vi "CD Init_Prepare Inline Data_Fill In RT part of Frame Descriptor -Broadcast.vi"(8 "RTs In":T1[](array[typedef]) {"Mode Codes"."Words Item Refs" format="%.0x"; "Mode Codes"."Words Block Data Refs"."Data Reference" format="%.0x"; "Mode Codes"."Timestamp Channel Data Reference" format="%.0x"; "subAddresses"."Words Item Refs" format="%.0x"; "subAddresses"."Words Block Data Refs"."Data Reference" format="%.0x"; "subAddresses"."Timestamp Channel Data Reference" format="%.0x"; "Status Channel Data Reference" format="%.0x"; "Command Channels Refs" format="%.0x"}, 11 "message":T10 {"Timestamp Channel Data Reference" format="%.0x"; "Status Channel Data Refs" format="%.0x"; "Words Item Refs" format="%.0x"; "Words Block Data Refs"."Data Reference" format="%.0x"}) -> (0 "RTs Out":T1[](array[typedef]) {"Mode Codes"."Words Item Refs" format="%.0x"; "Mode Codes"."Words Block Data Refs"."Data Reference" format="%.0x"; "Mode Codes"."Timestamp Channel Data Reference" format="%.0x"; "subAddresses"."Words Item Refs" format="%.0x"; "subAddresses"."Words Block Data Refs"."Data Reference" format="%.0x"; "subAddresses"."Timestamp Channel Data Reference" format="%.0x"; "Status Channel Data Reference" format="%.0x"; "Command Channels Refs" format="%.0x"}, 3 "RTs Frame Descriptors":T9[](array[typedef]) {"Status Channel Ref" format="%.0x"; "Words Block Data Refs"."Data Reference" format="%.0x"; "Timestamp Channel Data Reference" format="%.0x"})   [LabVIEW 2017, in "Ballard MIL-1553 Engine.lvlib"]
uses:
  Ballard MIL-1553 Engine.lvlib
  Shared/Controls and Global/RT Message.ctl
  Shared/Controls and Global/RT messageType.ctl
  Shared/Controls and Global/RT CWD1.ctl
  Shared/Controls and Global/RT CWD2.ctl
  <vilib>/NI Veristand/Custom Device API/Data Reference.ctl
  <vilib>/NI Veristand/Custom Device API/Custom Device Item Ref.ctl
  <vilib>/NI Veristand/Custom Device API/Block Data Reference.ctl
  Controls/RT Inline Frame Descriptor_RT.ctl
  Shared/Controls and Global/RT Remote Terminal.ctl
  Shared/Controls and Global/RT Remote Terminal_rtMode.ctl
  Shared/Controls and Global/RT Remote Terminal_RT subAddress.ctl
  Shared/Controls and Global/RT Remote Terminal_RT direction.ctl
  Shared/Controls and Global/RT Remote Terminal_RT Mode Code.ctl
  <vilib>/NI VeriStand/Custom Device API/Custom Device API.lvlib
  Shared/Ballard 1553 Shared.lvlib
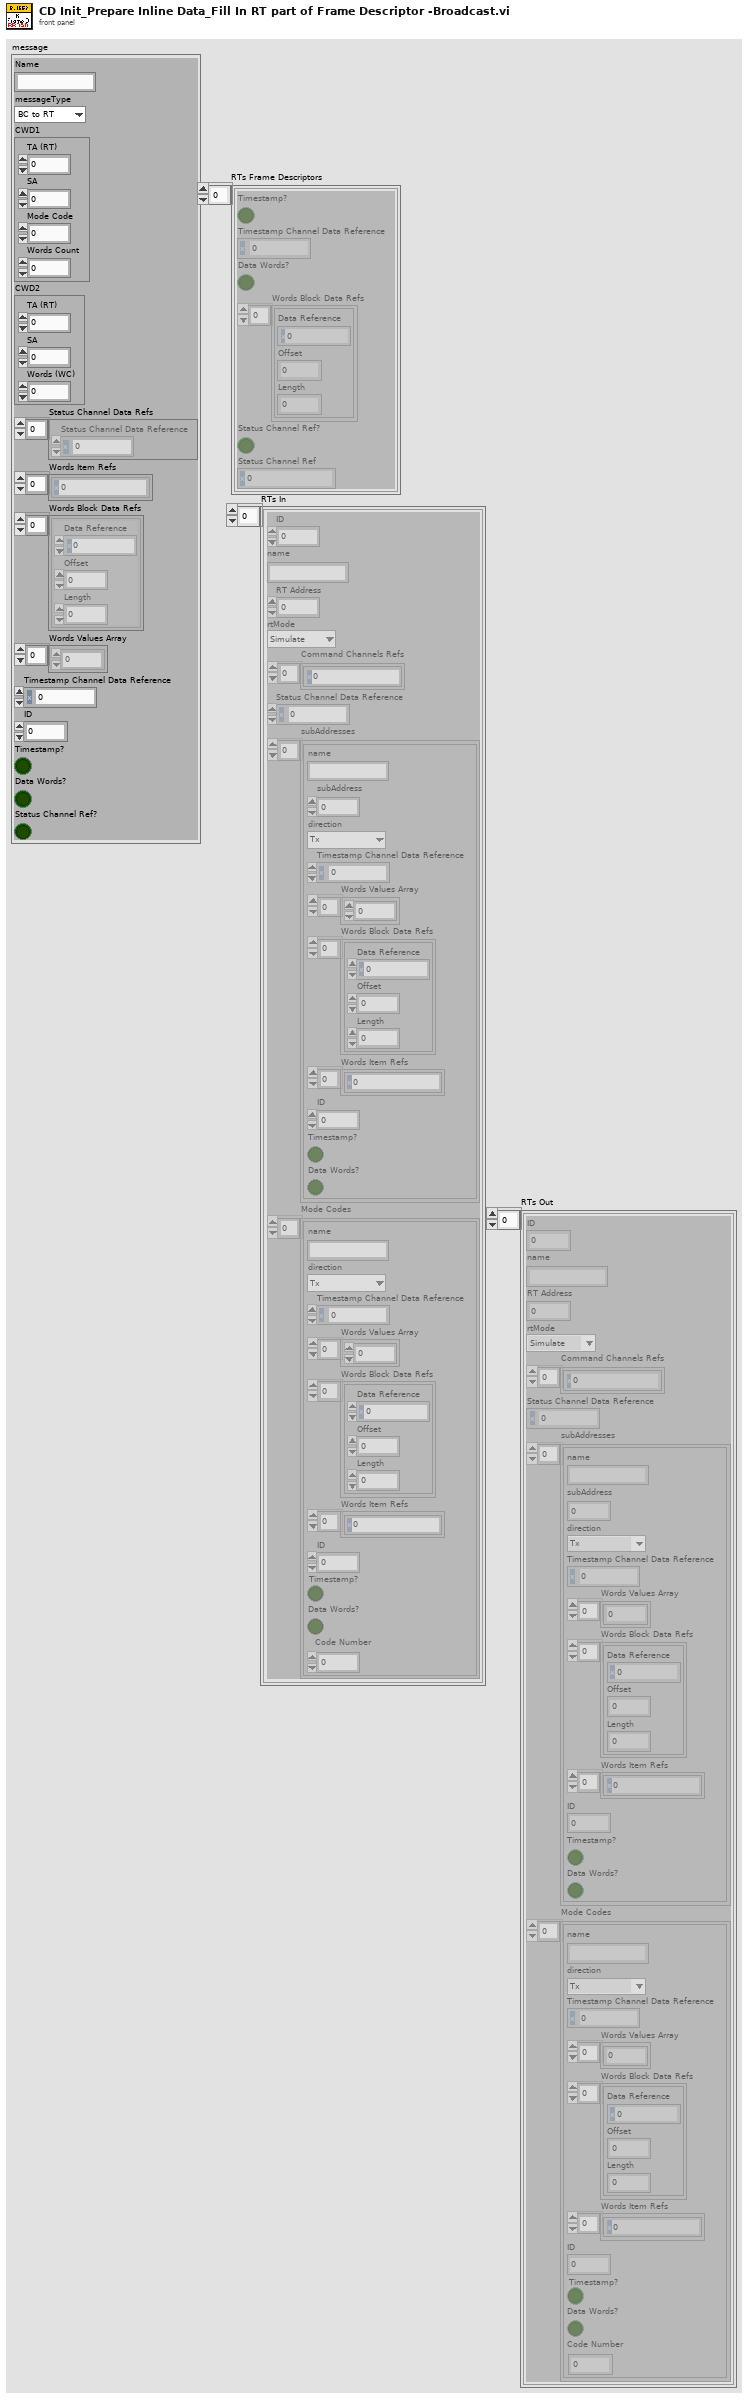
[diagram p1: front panel]
types:
  T1 = typedef "Ballard 1553 Shared.lvlib/RT Remote Terminal.ctl" = cluster{"ID":i32, "name":string, "RT Address":i32, "rtMode":T2, "Command Channels Refs":T3[], "Status Channel Data Reference":T4, "subAddresses":T5[], "Mode Codes":T8[]}
  T2 = typedef "Ballard 1553 Shared.lvlib/RT Remote Terminal_rtMode.ctl" = enum16{"Simulate", "Monitor", "Disable"}
  T3 = typedef "Custom Device API.lvlib/Custom Device Item Ref.ctl" = u64
  T4 = typedef "Custom Device API.lvlib/Data Reference.ctl" = i32
  T5 = typedef "Ballard 1553 Shared.lvlib/RT Remote Terminal_RT subAddress.ctl" = cluster{"name":string, "subAddress":i8, "direction":T6, "Timestamp Channel Data Reference":T4, "Words Values Array":u16[], "Words Block Data Refs":T7[], "Words Item Refs":T3[], "ID":i32, "Timestamp?":bool, "Data Words?":bool}
  T6 = typedef "Ballard 1553 Shared.lvlib/RT Remote Terminal_RT direction.ctl" = enum16{"Tx", "Rx"}
  T7 = typedef "Custom Device API.lvlib/Block Data Reference.ctl" = cluster{"Data Reference":T4, "Offset":u64, "Length":u64}
  T8 = typedef "Ballard 1553 Shared.lvlib/RT Remote Terminal_RT Mode Code.ctl" = cluster{"name":string, "direction":T6, "Timestamp Channel Data Reference":T4, "Words Values Array":u16[], "Words Block Data Refs":T7[], "Words Item Refs":T3[], "ID":i32, "Timestamp?":bool, "Data Words?":bool, "Code Number":i32}
  T9 = typedef "Ballard MIL-1553 Engine.lvlib/RT Inline Frame Descriptor_RT.ctl" = cluster{"Timestamp?":bool, "Timestamp Channel Data Reference":T4, "Data Words?":bool, "Words Block Data Refs":T7[], "Status Channel Ref?":bool, "Status Channel Ref":T3}
  T10 = typedef "Ballard 1553 Shared.lvlib/RT Message.ctl" = cluster{"Name":string, "messageType":T11, "CWD1":T12, "CWD2":T13, "Status Channel Data Refs":T4[], "Words Item Refs":T3[], "Words Block Data Refs":T7[], "Words Values Array":u16[], "Timestamp Channel Data Reference":T4, "ID":i32, "Timestamp?":bool, "Data Words?":bool, "Status Channel Ref?":bool}
  T11 = typedef "Ballard 1553 Shared.lvlib/RT messageType.ctl" = enum16{"BC to RT", "RT to BC", "RT to RT", "MC (Rx)", "MC (Tx)"}
  T12 = typedef "Ballard 1553 Shared.lvlib/RT CWD1.ctl" = cluster{"TA (RT)":i8, "SA":i8, "Mode Code":i8, "Words Count":i8}
  T13 = typedef "Ballard 1553 Shared.lvlib/RT CWD2.ctl" = cluster{"TA (RT)":i8, "SA":i8, "Words (WC)":i8}
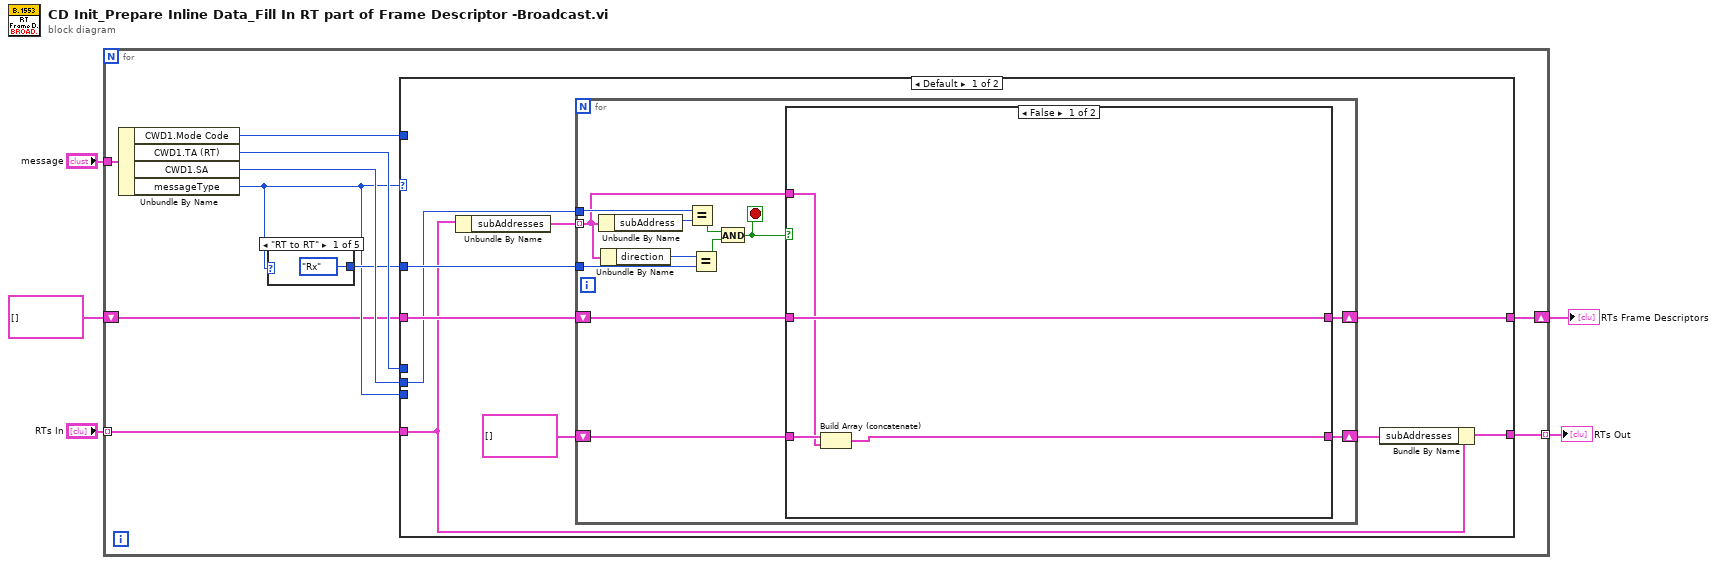
[diagram p0: block diagram]
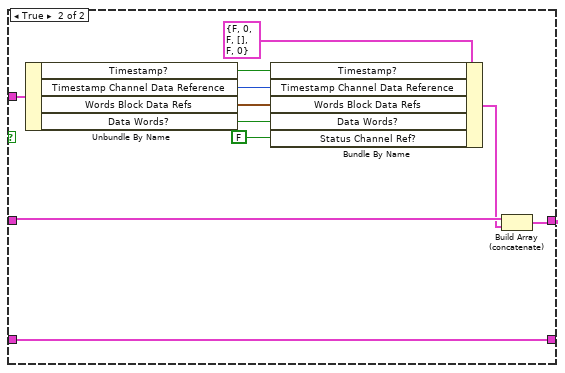
[diagram p2: hidden frame]
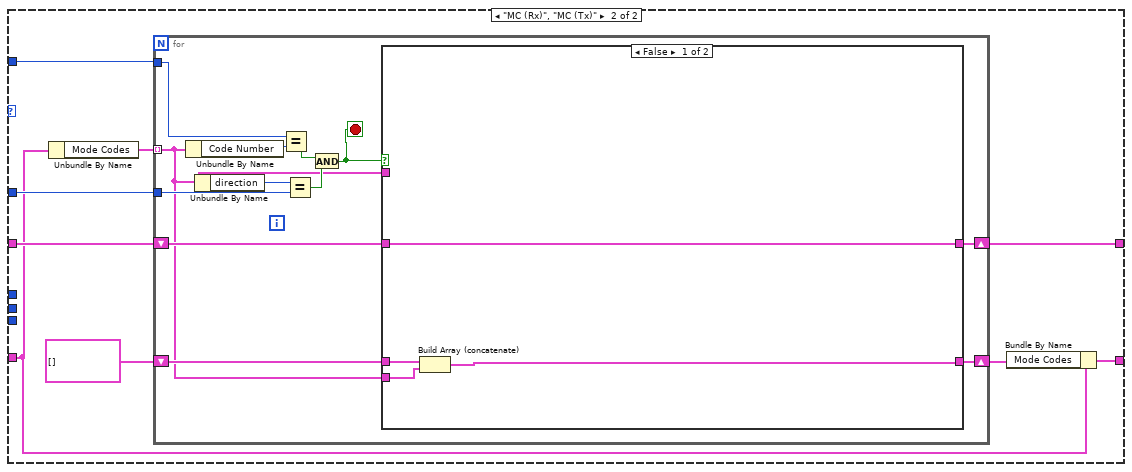
[diagram p3: hidden frame]
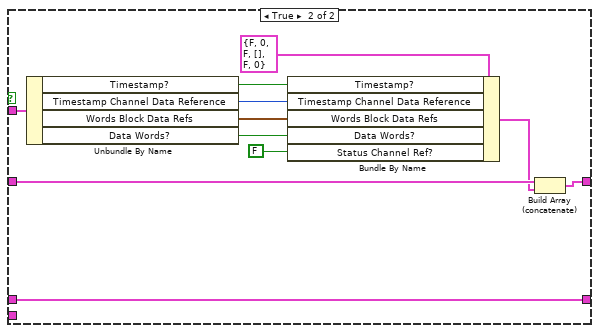
[diagram p4: hidden frame]
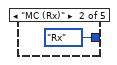
[diagram p5: hidden frame]
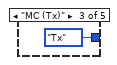
[diagram p6: hidden frame]
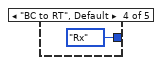
[diagram p7: hidden frame]
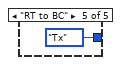
[diagram p8: hidden frame]
diagram:
  n1 = for {
    tunnel: "message" -> [w13]
    tunnel: "RTs In" -> [w12] mode=indexing
    shift-right: [w7] -> w2
    shift-left: T9[] [] -> [w8]
    tunnel: [w6] -> w1 mode=indexing
    n2 = Unbundle By Name(w13) -> ("CWD1.Mode Code"=w9:i8, "CWD1.TA (RT)"=w15:i8, "CWD1.SA"=w14:i8, "messageType"=w10:T11)
    n3 = case shown="\"RT to RT\"" w10 {
      tunnel: [RT_Remote_Terminal_RT_direction."Rx" ("y") RT_Remote_Terminal_RT_direction."Rx" ("y") RT_Remote_Terminal_RT_direction."Tx" ("y") RT_Remote_Terminal_RT_direction."Rx" ("y") RT_Remote_Terminal_RT_direction."Tx" ("y")] -> w11
      frame "RT to RT" {
      }
      frame "MC (Rx)" {
      }
      frame "MC (Tx)" {
      }
      frame "BC to RT", Default {
      }
      frame "RT to BC" {
      }
    }
    n4 = case shown="Default" w10 {
      tunnel: w15 -> [_ _]
      tunnel: w14 -> [w20 _]
      tunnel: w12 -> [w18 w54]
      tunnel: w11 -> [w24 w60]
      tunnel: w10 -> [_ _]
      tunnel: w9 -> [_ w59]
      tunnel: w8 -> [w22 w57]
      tunnel: [w21 w56] -> w7
      tunnel: [w17 w52] -> w6
      frame Default {
        n5 = Unbundle By Name(w18) -> ("subAddresses"=w23:T5[])
        n6 = for {
          tunnel: w23 -> [w29] mode=indexing
          tunnel: w20 -> [w36]
          tunnel: w24 -> [w31]
          shift-right: [w27] -> w21
          shift-left: w22 -> [w28]
          shift-right: [w25] -> w16
          shift-left: T5[] [] -> [w26]
          stop <- w30 stop-if-true
          n7 = Unbundle By Name(w29) -> ("subAddress"=w35:i8)
          n8 = Unbundle By Name(w29) -> ("direction"=w34:T6)
          n9 = Equal?(x=w36, y=w35) -> (x = y?=w33:bool)
          n10 = Equal?(x=w34, y=w31) -> (x = y?=w32:bool)
          n11 = And(x=w33, y=w32) -> (x .and. y?=w30:bool)
          n12 = case shown="False" w30 {
            tunnel: w29 -> [w38 w46]
            tunnel: w28 -> [w40 w45]
            tunnel: [w40 w43] -> w27
            tunnel: w26 -> [w39 w41]
            tunnel: [w37 w41] -> w25
            frame False {
              n13 = Build Array (concatenate)(w39, w38) -> (w37:T5[])
            }
            frame True {
              n14 = Unbundle By Name(w46) -> ("Timestamp?"=w42:bool, "Timestamp Channel Data Reference"=w50:T4, "Words Block Data Refs"=w51:T7[], "Data Words?"=w49:bool)
              n15 = Bundle By Name(cluster=T9 {"Timestamp?"=FALSE, "Timestamp Channel Data Reference"=0, "Data Words?"=FALSE, "Words Block Data Refs"=[], "Status Channel Ref?"=FALSE, "Status Channel Ref"=0} ("RT"), "Timestamp?"=w42, "Timestamp Channel Data Reference"=w50, "Words Block Data Refs"=w51, "Data Words?"=w49, "Status Channel Ref?"=FALSE) -> (w44:T9)
              n16 = Build Array (concatenate)(w45, w44) -> (w43:T9[])
            }
          }
        }
        n17 = Bundle By Name(cluster=w18, "subAddresses"=w16) -> (w17:T1)
      }
      frame "MC (Rx)", "MC (Tx)" {
        n18 = Unbundle By Name(w54) -> ("Mode Codes"=w58:T8[])
        n19 = for {
          tunnel: w58 -> [w62] mode=indexing
          tunnel: w59 -> [w72]
          tunnel: w60 -> [w67]
          shift-right: [w64] -> w56
          shift-left: w57 -> [w65]
          shift-right: [w61] -> w53
          shift-left: T8[] [] -> [w63]
          stop <- w66 stop-if-true
          n20 = Unbundle By Name(w62) -> ("Code Number"=w71:i32)
          n21 = Unbundle By Name(w62) -> ("direction"=w70:T6)
          n22 = Equal?(x=w72, y=w71) -> (x = y?=w69:bool)
          n23 = Equal?(x=w70, y=w67) -> (x = y?=w68:bool)
          n24 = And(x=w69, y=w68) -> (x .and. y?=w66:bool)
          n25 = case shown="False" w66 {
            tunnel: w65 -> [w76 w80]
            tunnel: [w76 w78] -> w64
            tunnel: w62 -> [_ w81]
            tunnel: w63 -> [w75 w77]
            tunnel: w62 -> [w74 _]
            tunnel: [w73 w77] -> w61
            frame False {
              n26 = Build Array (concatenate)(w75, w74) -> (w73:T8[])
            }
            frame True {
              n27 = Unbundle By Name(w81) -> ("Timestamp?"=w84:bool, "Timestamp Channel Data Reference"=w86:T4, "Words Block Data Refs"=w87:T7[], "Data Words?"=w85:bool)
              n28 = Bundle By Name(cluster=T9 {"Timestamp?"=FALSE, "Timestamp Channel Data Reference"=0, "Data Words?"=FALSE, "Words Block Data Refs"=[], "Status Channel Ref?"=FALSE, "Status Channel Ref"=0} ("RT"), "Timestamp?"=w84, "Timestamp Channel Data Reference"=w86, "Words Block Data Refs"=w87, "Data Words?"=w85, "Status Channel Ref?"=FALSE) -> (w79:T9)
              n29 = Build Array (concatenate)(w80, w79) -> (w78:T9[])
            }
          }
        }
        n30 = Bundle By Name(cluster=w54, "Mode Codes"=w53) -> (w52:T1)
      }
    }
  }
  "RTs Frame Descriptors" <- w2
  "RTs Out" <- w1
